vi "Launch Nested Actors.vi"(8 "error in (no error)":errorcluster, 11 "ATM Controller in":refnum<class "ATM Controller.lvclass">) -> (0 "error out":errorcluster, 3 "ATM Controller out":refnum<class "ATM Controller.lvclass">)   [LabVIEW 2019, in "ATM Controller.lvlib" / "ATM Controller.lvclass"]
uses:
  ATM Controller.lvclass
  C:/Program Files (x86)/National Instruments/LabVIEW 2019/vi.lib/ActorFramework/Actor/Actor.lvclass
  Simulated User Console Actor/Simulated User Console Actor/Simulated User Console Actor.lvclass
  Simulated Display Console Actor/Simulated User Console Actor/Simulated Display Console Actor.lvclass
  Simulated Sensor Interface Actor/Simulated User Console Actor/Simulated Sensor Interface Actor.lvclass
  Simulated Configuration Database Actor/Simulated Configuration Database Actor/Configuration Database Actor.lvclass
  ATM Controller.lvclass/ATM Controller.ctl
  <vilib>/ActorFramework/Actor/Actor.lvclass
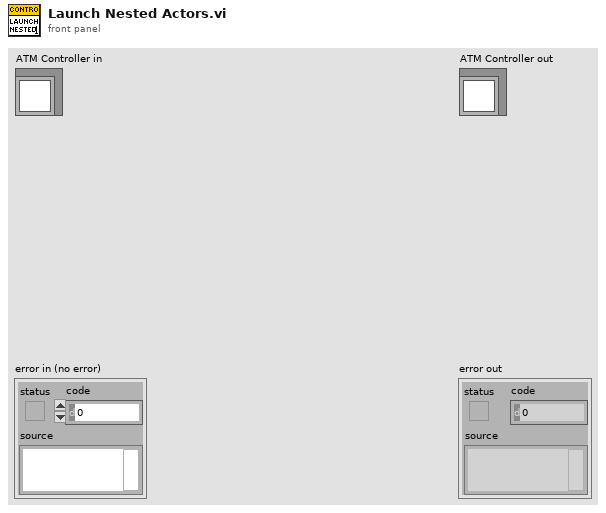
[diagram p1: front panel]
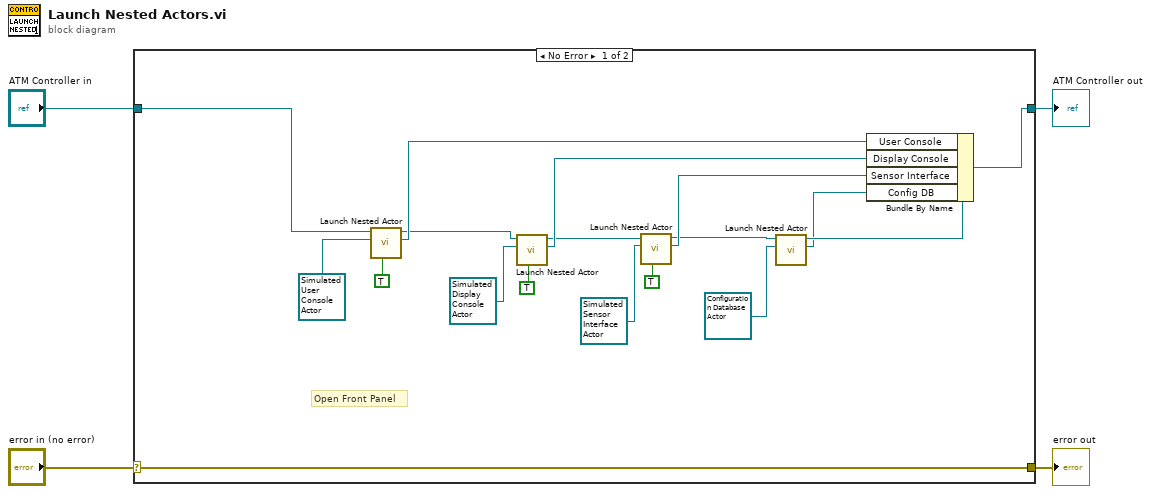
[diagram p0: block diagram]
diagram:
  n1 = case shown="No Error" "error in (no error)" {
    selector: "error in (no error)" -> [w22 w24]
    tunnel: [w22 w24] -> w3
    tunnel: [w20 w23] -> w1
    tunnel: "ATM Controller in" -> [w21 w23]
    frame No Error {
      # "Open Front Panel"
      n2 = call <vilib>:"Launch Nested Actor.vi"("Open Actor Core front panel? (F)"=TRUE, "Nested Actor"=refnum<class "Simulated User Console Actor.lvclass"> refnum ("Simulated User Console Actor.lvlib:Simulated User Console Actor.lvclass"), "Caller Actor in"=w21) -> ("Nested Actor's Enqueuer"=w18:refnum<class "Message Enqueuer.lvclass">, "Caller Actor out"=w17:refnum<class "ATM Controller.lvclass">)  [unwired: 6 in, 1 out]
      n3 = call <vilib>:"Launch Nested Actor.vi"("Open Actor Core front panel? (F)"=TRUE, "Nested Actor"=refnum<class "Simulated Display Console Actor.lvclass"> refnum ("Simulated Display Console Actor.lvlib:Simulated Display Console Actor.lvclass"), "Caller Actor in"=w17) -> ("Nested Actor's Enqueuer"=w14:refnum<class "Message Enqueuer.lvclass">, "Caller Actor out"=w12:refnum<class "ATM Controller.lvclass">)  [unwired: 6 in, 1 out]
      n4 = call <vilib>:"Launch Nested Actor.vi"("Open Actor Core front panel? (F)"=TRUE, "Nested Actor"=refnum<class "Simulated Sensor Interface Actor.lvclass"> refnum ("Simulated Sensor Interface Actor.lvlib:Simulated Sensor Interface Actor.lvclass"), "Caller Actor in"=w12) -> ("Nested Actor's Enqueuer"=w10:refnum<class "Message Enqueuer.lvclass">, "Caller Actor out"=w8:refnum<class "ATM Controller.lvclass">)  [unwired: 6 in, 1 out]
      n5 = call <vilib>:"Launch Nested Actor.vi"("Nested Actor"=refnum<class "Configuration Database Actor.lvclass"> refnum ("Simulated Configuration Database Actor.lvlib:Simulated Configuration Database Actor.lvclass"), "Caller Actor in"=w8) -> ("Nested Actor's Enqueuer"=w5:refnum<class "Message Enqueuer.lvclass">, "Caller Actor out"=w7:refnum<class "ATM Controller.lvclass">)  [unwired: 7 in, 1 out]
      n6 = Bundle By Name(cluster=w7, "User Console"=w18, "Display Console"=w14, "Sensor Interface"=w10, "Config DB"=w5) -> (w20:refnum<class "ATM Controller.lvclass">)
    }
    frame Error {
    }
  }
  "error out" <- w3
  "ATM Controller out" <- w1
